vi "Motor Current to encoder.vi"(9 "Drive Motor current":dbl) -> (1 "Encoder velocity":dbl)   [LabVIEW 2017]
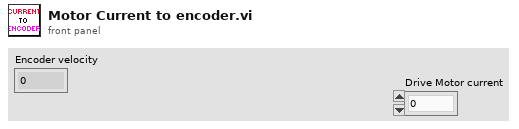
[diagram p1: front panel]
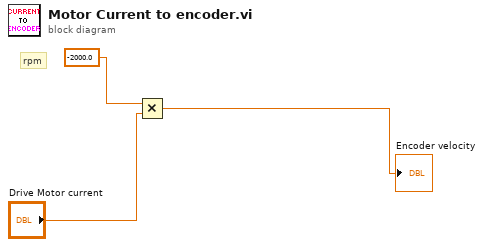
[diagram p0: block diagram]
diagram:
  # "rpm"
  n1 = Multiply(x=-2000.0, y="Drive Motor current") -> (x*y=→"Encoder velocity":dbl)
